vi "Watchdog Check.vi"(8 "error in (no error)":errorcluster, 11 "Timeout (ms)":u32) -> (0 "error out":errorcluster, 1 "Timed Out Watchdog":i32, 2 "Skipped?":bool=TRUE, 3 "Timeout?":bool)   [LabVIEW 2014, in "RT Watchdog.lvlib"]
uses:
  RT Watchdog.lvlib
  Watchdog actions.ctl
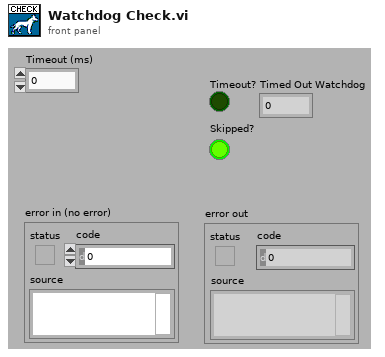
[diagram p1: front panel]
types:
  T1 = typedef "RT Watchdog.lvlib/Watchdog actions.ctl" = enum16{"Init", "Enable", "Service", "Disable", "Check"}
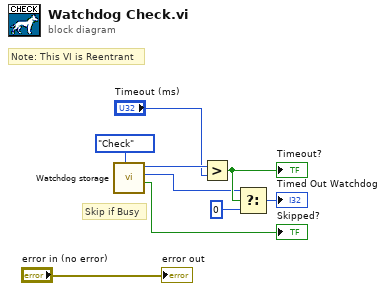
[diagram p0: block diagram]
diagram:
  # "Skip if Busy"
  # "Note: This VI is Reentrant"
  n1 = call "Watchdog storage.vi"("Command"=Watchdog_actions."Check") -> ("Skipped?"=→"Skipped?":bool, "Max index"=w2:i32, "Max Time"=w7:u32)  [unwired: 8 in]
  n2 = Greater?(x=w7, y="Timeout (ms)") -> (0:w4:bool)
  "Timeout?" <- w4
  n3 = Select(t=w2, s=w4, f=0) -> (s? t:f=→"Timed Out Watchdog":i32)
  "error out" <- "error in (no error)"
